vi "数据回放.vi"(8 "Error":errorcluster) -> (0 "Error out":errorcluster)   [LabVIEW 2011]
panel:
  out "units":string[](array[string])
  in  "Temp chart":waveform(dbl)
  in  "T":T1={"Error"={"status"=FALSE, "code"=0, "source"=""}, "Test Info"={"Test Name"="", "Tester"=""}, "test data"=[{"t0"=timestamp(0 s since 1904-01-01), "dt"=1.0, "Y"=[]}, {"t0"=timestamp(0 s since 1904-01-01), "dt"=1.0, "Y"=[]}, {"t0"=timestamp(0 s since 1904-01-01), "dt"=1.0, "Y"=[]}, {"t0"=timestamp(0 s since 1904-01-01), "dt"=0.001, "Y"=[]}], "Index Vibration Waveform"={"t0"=timestamp(0 s since 1904-01-01), "dt"=1.0, "Y"=[]}, "report information"={"Test Info"={"Test Name"="", "Tester"=""}, "temp chart 2"=refnum, "P chart 2"=refnum}, "TdmsInfo"={"Read Chan Name"="", "Vibr Chn Name"=[], "Read Group Name"="", "Vibr Group Name"=[]}}
  in  "选项卡控件":enum32{"选项卡 1", "选项卡 2"}(tab)
  in  "temp chart":dbl[](graph)
  in  "P chart":dbl[](graph)
  in  "Tree":string(tree)="PXI-4472/ai0"
  in  "Exit":bool caption="返回"
  in  "Report":bool caption="生成报表"
  in  "Open":bool caption="读取"
  out "Tester":string caption="实验人"
  out "Test Name":string caption="实验名称"
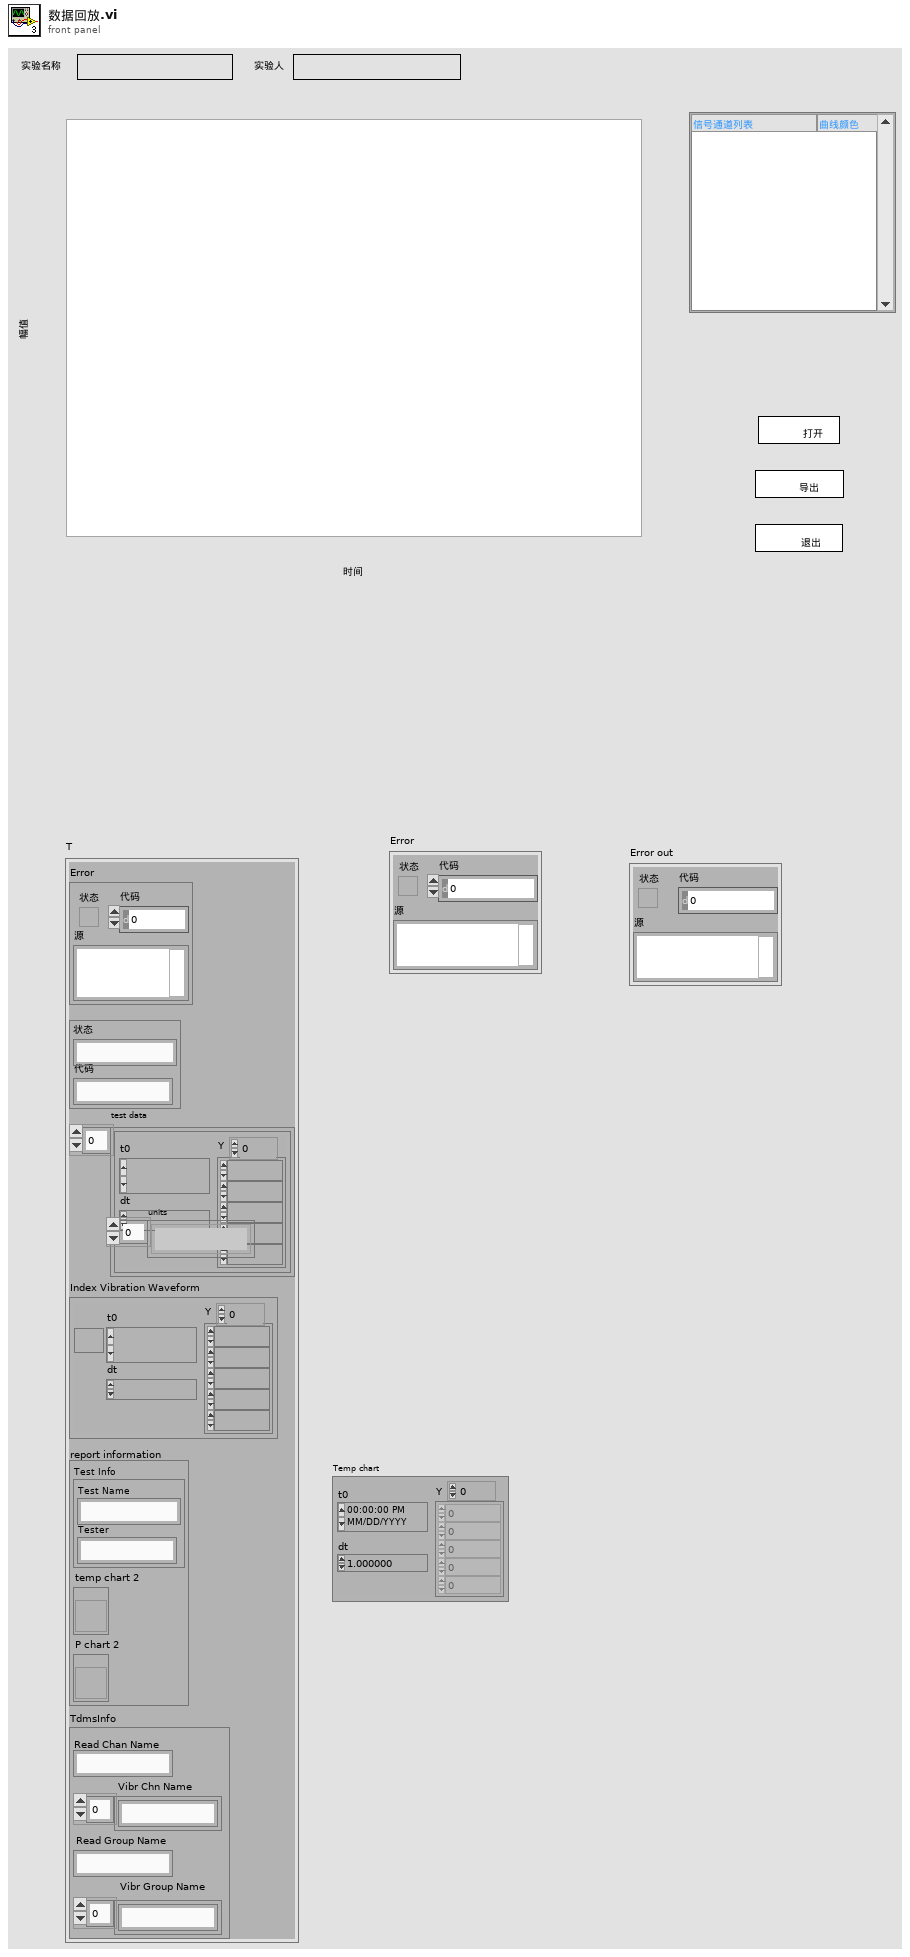
[diagram p1: front panel]
types:
  T1 = typedef "数据回放蔟0.ctl" = cluster{"Error":errorcluster, "Test Info":cluster{"Test Name":string, "Tester":string}, "test data":waveform(dbl)[], "Index Vibration Waveform":waveform(dbl), "report information":cluster{"Test Info":cluster{"Test Name":string, "Tester":string}, "temp chart 2":refnum<vi>, "P chart 2":refnum<vi>}, "TdmsInfo":cluster{"Read Chan Name":string, "Vibr Chn Name":string[], "Read Group Name":string, "Vibr Group Name":string[]}}
  T2 = typedef "Enum Query_Ctrls-某型振动实验台测试系统.ctl" = enum16{"Initialize", "No Action", "Open TDMS File", "Read Raw Data", "Analyze Data", "Display Data", "Generate Report", "computer timer", "Error Handle", "Exit"}
  T3 = typedef "Enum File IO - FGV(V)_Ctrls-某型振动实验台测试系统.ctl" = enum16{"New", "Open", "Write Info", "Write Data", "Read Info", "Read Chan Names", "Read Data", "Close", "None"}
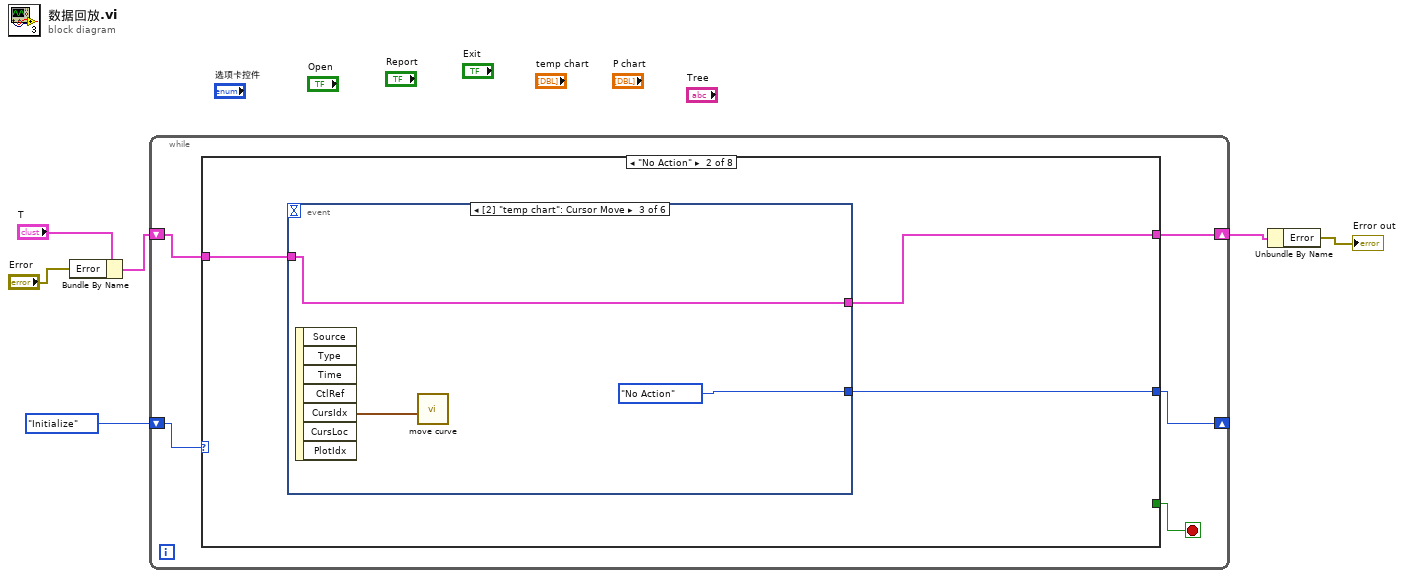
[diagram p0: block diagram]
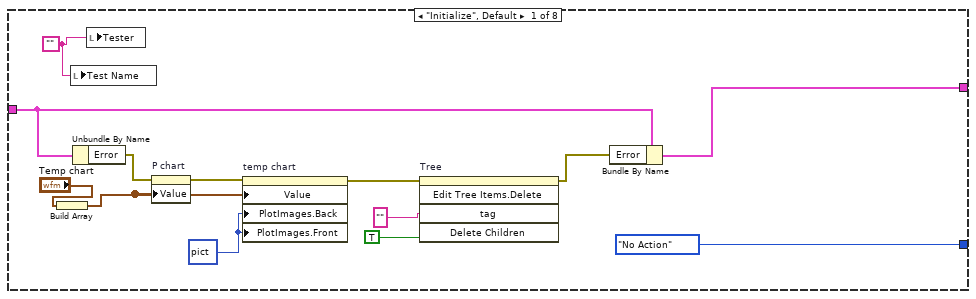
[diagram p2: hidden frame]
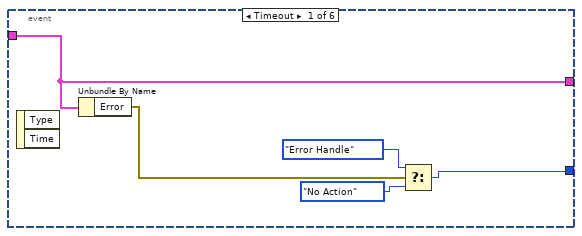
[diagram p3: hidden frame]
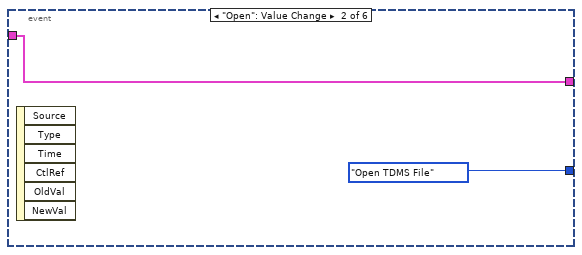
[diagram p4: hidden frame]
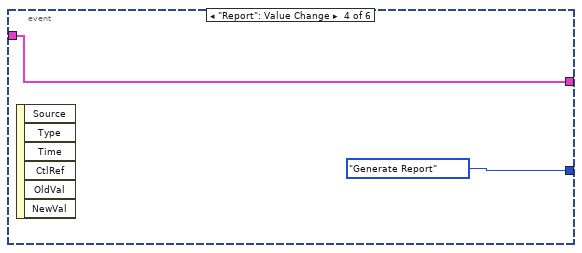
[diagram p5: hidden frame]
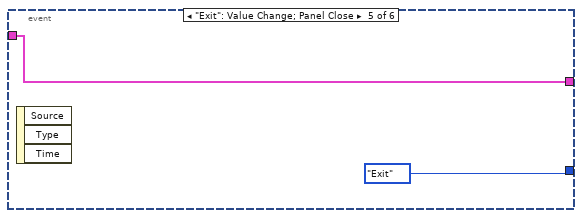
[diagram p6: hidden frame]
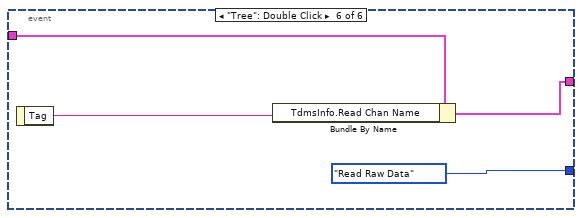
[diagram p7: hidden frame]
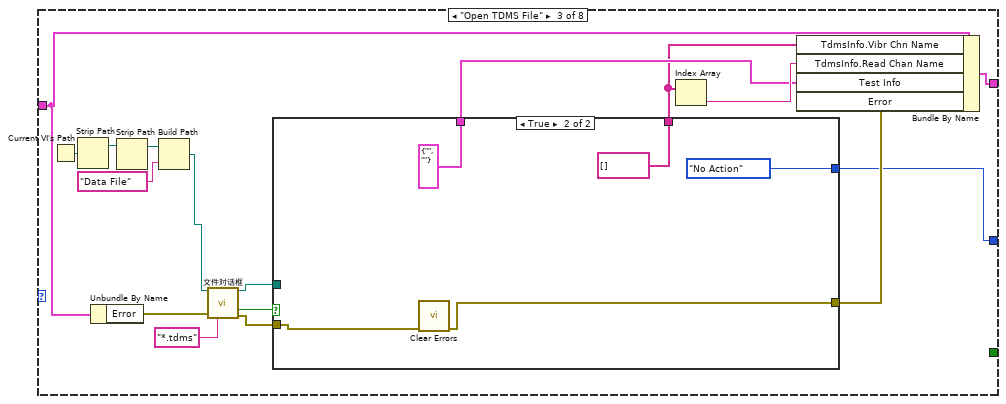
[diagram p8: hidden frame]
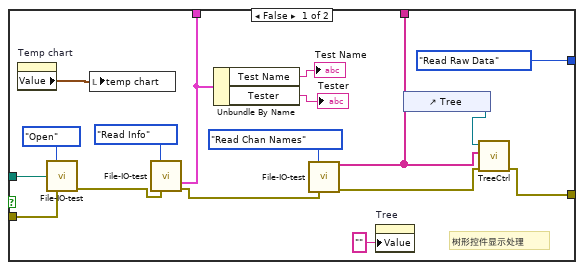
[diagram p9: hidden frame]
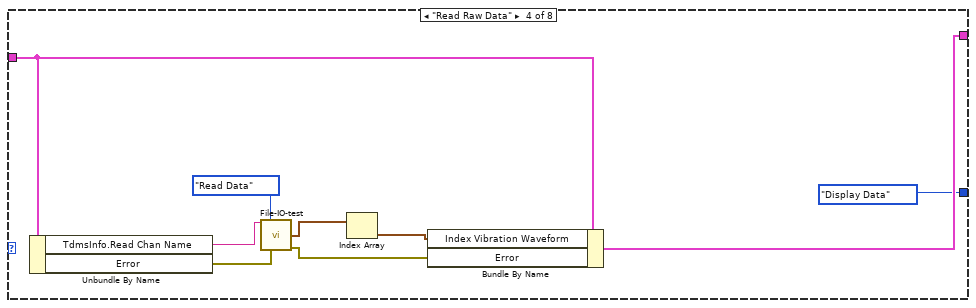
[diagram p10: hidden frame]
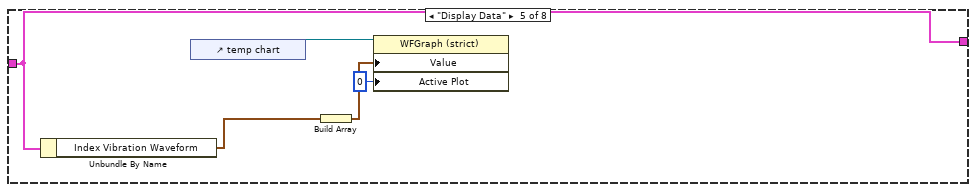
[diagram p11: hidden frame]
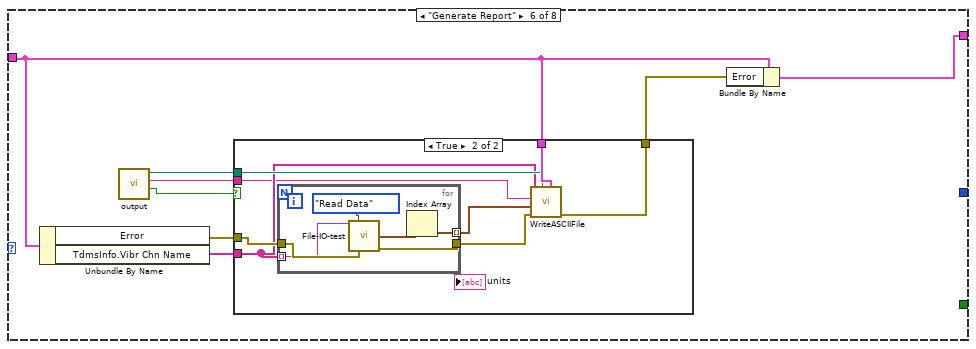
[diagram p12: hidden frame]
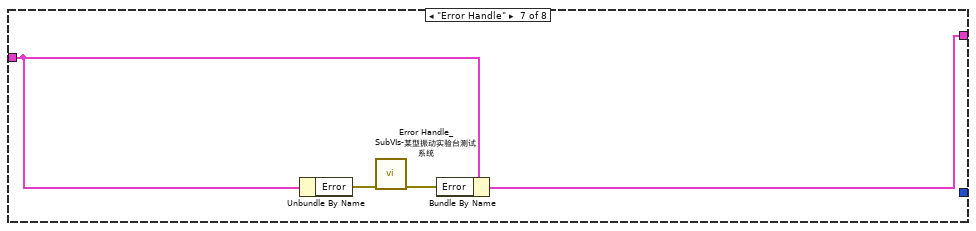
[diagram p14: hidden frame]
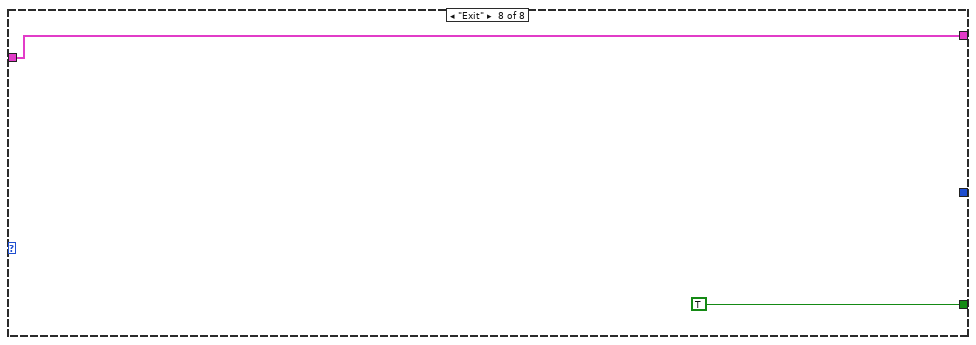
[diagram p15: hidden frame]
diagram:
  n1 = Bundle By Name(cluster="T", "Error"="Error") -> (w1:T1)
  n2 = while {
    shift-right: [w11] -> _
    shift-left: Enum_Query_Ctrls-某型振动实验台测试系统."Initialize" ("Enum") -> [w10]
    shift-right: [w8] -> w5
    shift-left: w1 -> [w9]
    stop <- w7 stop-if-true
    n3 = case shown="\"No Action\"" w10 {
      tunnel: [Enum_Query_Ctrls-某型振动实验台测试系统."No Action" ("Enum") w27 w46 Enum_Query_Ctrls-某型振动实验台测试系统."Display Data" ("Enum") _ _ _ _] -> w11
      tunnel: w9 -> [w15 w26 w52 w90 w94 w99 w122 w125]
      tunnel: [w14 w25 w51 w88 w94 w100 w121 w125] -> w8
      tunnel: [_ _ _ _ _ _ _ TRUE] -> w7
      frame "Initialize", Default {
        w20 = picture data[5B] ("曲线图像:前景")
        w24 = ""
        n4 = Build Array("Temp chart") -> (w19:waveform(dbl)[])
        n5 = local write "Test Name"(w24) -> ()
        n6 = Unbundle By Name(w15) -> ("Error"=w18:errorcluster)
        n7 = local write "Tester"(w24) -> ()
        n8 = property on="P chart" class="WFGraph (strict)"(error in=w18, "Value"=w19) -> (error out=w17:errorcluster)  [unwired: 1 in, 1 out]
        n9 = property on="temp chart" class="WFGraph (strict)"(error in=w17, "Value"=w19, "PlotImages.Back"=w20, "PlotImages.Front"=w20) -> (error out=w16:errorcluster)  [unwired: 1 in, 1 out]
        n10 = invoke on="Tree" class="Tree (严格)" method="Edit Tree Items.Delete"(error in=w16, "tag"="" ("Tag"), "Delete Children"=TRUE ("Delete Children?")) -> (error out=w13:errorcluster)  [unwired: 2 in, 4 out]
        n11 = Bundle By Name(cluster=w15, "Error"=w13) -> (w14:T1)
      }
      frame "No Action" {
        n12 = event shown="[2] \"temp chart\": Cursor Move" {
          selector: _ -> [_ _ _ _ _ _]
          dyn-events: _ -> [_ _ _ _ _ _]
          timeout: _ -> [_ _ _ _ _ _]
          tunnel: [w30 Enum_Query_Ctrls-某型振动实验台测试系统."Open TDMS File" ("Enum") Enum_Query_Ctrls-某型振动实验台测试系统."No Action" ("Enum") Enum_Query_Ctrls-某型振动实验台测试系统."Generate Report" ("Enum") Enum_Query_Ctrls-某型振动实验台测试系统."Exit" ("Enum") Enum_Query_Ctrls-某型振动实验台测试系统."Read Raw Data" ("Enum")] -> w27
          tunnel: w26 -> [w28 w33 w35 w38 w40 w43]
          tunnel: [w28 w33 w35 w38 w40 w42] -> w25
          event Timeout {
            n13 = event-data() -> ()  [unwired: 3 out]
            n14 = Unbundle By Name(w28) -> ("Error"=w29:errorcluster)
            n15 = Select(t=Enum_Query_Ctrls-某型振动实验台测试系统."Error Handle" ("Enum"), s=w29, f=Enum_Query_Ctrls-某型振动实验台测试系统."No Action" ("Enum")) -> (s? t:f=w30:T2)
          }
          event "Open": Value Change {
            n16 = event-data() -> ()  [unwired: 7 out]
          }
          event "temp chart": Cursor Move {
            n17 = event-data() -> ("CursLoc"=w36:cluster{"X":dbl, "Y":dbl})  [unwired: 7 out]
            n18 = call "move curve.vi"("XY"=w36) -> ()  [unwired: 2 in, 9 out]
          }
          event "Report": Value Change {
            n19 = event-data() -> ()  [unwired: 7 out]
          }
          event "Exit": Value Change; Panel Close {
            n20 = event-data() -> ()  [unwired: 4 out]
          }
          event "Tree": Double Click {
            n21 = event-data() -> ("Tag"=w45:string)  [unwired: 1 out]
            n22 = Bundle By Name(cluster=w43, "TdmsInfo.Read Chan Name"=w45) -> (w42:T1)
          }
        }
      }
      frame "Open TDMS File" {
        n23 = Current VI's Path() -> (path=w61:path)
        n24 = Strip Path(path=w61) -> (stripped path=w62:path)  [unwired: 1 out]
        n25 = Unbundle By Name(w52) -> ("Error"=w57:errorcluster)
        n26 = Strip Path(path=w62) -> (stripped path=w60:path)  [unwired: 1 out]
        n27 = Build Path(base path=w60, name or relative path="Data File") -> (appended path=w56:path)
        n28 = call "文件对话框"("start path"=w56, "error in"=w57, "pattern (all files)"="*.tdms") -> ("selected path"=w55:path, "cancelled"=w53:bool, "error out"=w54:errorcluster)  [unwired: 4 in, 6 out]
        n29 = case shown="True" w53 {
          tunnel: w55 -> [w76 _]
          tunnel: [w74 cluster{"Test Name":string, "Tester":string} {"Test Name"="", "Tester"=""} ("Name")] -> w49
          tunnel: w54 -> [w69 w82]
          tunnel: [w65 string[] [] ("Vibration Channel Name Output")] -> w48
          tunnel: [w63 w81] -> w47
          tunnel: [Enum_Query_Ctrls-某型振动实验台测试系统."Read Raw Data" ("Enum") Enum_Query_Ctrls-某型振动实验台测试系统."No Action" ("Enum")] -> w46
          frame False {
            # "树形控件显示处理"
            n30 = property on="Temp chart" class="WFD (strict)"() -> ("Value"=w78:waveform(dbl))  [unwired: 2 in, 2 out]
            n31 = call "File-IO-test.vi"("Operation"=Enum_File_IO_-_FGV(V)_Ctrls-某型振动实验台测试系统."Open", "文件路径"=w76, "error in"=w69) -> ("error out"=w75:errorcluster)  [unwired: 9 in, 3 out]
            n32 = local write "temp chart"(w78) -> ()
            n33 = call "File-IO-test.vi"("Operation"=Enum_File_IO_-_FGV(V)_Ctrls-某型振动实验台测试系统."Read Info", "error in"=w75) -> ("Test Info 2"=w74:cluster{"Test Name":string, "Tester":string}, "error out"=w71:errorcluster)  [unwired: 10 in, 2 out]
            n34 = Unbundle By Name(w74) -> ("Test Name"=→"Test Name":string, "Tester"=→"Tester":string)
            n35 = call "File-IO-test.vi"("Operation"=Enum_File_IO_-_FGV(V)_Ctrls-某型振动实验台测试系统."Read Chan Names", "error in"=w71) -> ("通道名"=w65:string[], "error out"=w64:errorcluster)  [unwired: 10 in, 2 out]
            n36 = property on="Tree" class="Tree (strict)"("Value"="" ("Tree")) -> ()  [unwired: 2 in, 2 out]
            n37 = control-ref of="Tree"() -> (w66:refnum<vi>)
            n38 = call "TreeCtrl.vi"("错误输入（无错误）"=w64, "Vibration Channel Name"=w65, "Tree in"=w66) -> ("错误输出"=w63:errorcluster)  [unwired: 8 in]
          }
          frame True {
            n39 = call <vilib>:"Clear Errors.vi"("error in (no error)"=w82) -> ("error out"=w81:errorcluster)  [unwired: 6 out]
          }
        }
        n40 = Index Array(array=w48) -> (element=w50:string)  [unwired: 1 in]
        n41 = Bundle By Name(cluster=w52, "TdmsInfo.Vibr Chn Name"=w48, "TdmsInfo.Read Chan Name"=w50, "Test Info"=w49, "Error"=w47) -> (w51:T1)
      }
      frame "Read Raw Data" {
        n42 = Unbundle By Name(w90) -> ("TdmsInfo.Read Chan Name"=w85:string, "Error"=w92:errorcluster)
        n43 = call "File-IO-test.vi"("Chan"=w85, "Operation"=Enum_File_IO_-_FGV(V)_Ctrls-某型振动实验台测试系统."Read Data", "error in"=w92) -> ("Vibration Waveform out"=w91:waveform(dbl)[], "error out"=w86:errorcluster)  [unwired: 9 in, 2 out]
        n44 = Index Array(array=w91) -> (element=w89:waveform(dbl))  [unwired: 1 in]
        n45 = Bundle By Name(cluster=w90, "Index Vibration Waveform"=w89, "Error"=w86) -> (w88:T1)
      }
      frame "Display Data" {
        n46 = Unbundle By Name(w94) -> ("Index Vibration Waveform"=w95:waveform(dbl))
        n47 = control-ref of="temp chart"() -> (w97:refnum<vi>)
        n48 = Build Array(w95) -> (w98:waveform(dbl)[])
        n49 = property class="WFGraph (strict)"(reference=w97, "Value"=w98, "Active Plot"=u32 0 ("活动曲线")) -> ()  [unwired: 1 in, 2 out]
      }
      frame "Generate Report" {
        n50 = Unbundle By Name(w99) -> ("Error"=w106:errorcluster, "TdmsInfo.Vibr Chn Name"=w103:string[])
        n51 = call "output.vi"() -> ("ok?"=w101:bool, "txt?excel"=w104:string, "path"=w105:path)  [unwired: 9 out]
        n52 = case shown="True" w101 {
          tunnel: w106 -> [_ w114]
          tunnel: w105 -> [_ w112]
          tunnel: w104 -> [_ w110]
          tunnel: w103 -> [_ w111]
          tunnel: [_ w107] -> w102
          tunnel: w99 -> [_ w113]
          frame False {
          }
          frame True {
            n53 = for {
              tunnel: w111 -> [w115] mode=indexing
              tunnel: [w118] -> w109 mode=indexing
              tunnel: w114 -> [w116]
              tunnel: [w117] -> w108
              n54 = call "File-IO-test.vi"("Chan"=w115, "Operation"=Enum_File_IO_-_FGV(V)_Ctrls-某型振动实验台测试系统."Read Data", "error in"=w116) -> ("Vibration Waveform out"=w119:waveform(dbl)[], "error out"=w117:errorcluster)  [unwired: 9 in, 2 out]
              n55 = Index Array(array=w119) -> (element=w118:waveform(dbl))  [unwired: 1 in]
            }
            n56 = call "WriteASCIIFile.vi"("T"=w113, "file (use dialog)"=w112, "error in (no error)"=w108, "data"=w109, "格式"=w110, "chanel name"=w111) -> ("error out"=w107:errorcluster)  [unwired: 5 in]
          }
        }
        n57 = Bundle By Name(cluster=w99, "Error"=w102) -> (w100:T1)
      }
      frame "Error Handle" {
        n58 = Unbundle By Name(w122) -> ("Error"=w124:errorcluster)
        n59 = call "Error Handle_SubVIs-某型振动实验台测试系统.vi"("error in"=w124) -> ("error out"=w123:errorcluster)  [unwired: 10 out]
        n60 = Bundle By Name(cluster=w122, "Error"=w123) -> (w121:T1)
      }
      frame "Exit" {
      }
    }
  }
  n61 = Unbundle By Name(w5) -> ("Error"=→"Error out":errorcluster)
